vi "Skipback_171213.vi"(6 "Y out 3":i32[](array[numeric]), 9 "X in":i32[](array[numeric]), 10 "Skip Back Button":bool, 11 "Boolean in":refnum<vi>) -> (2 "Y out":i32[](array[numeric]), 3 "Y out 2":i32[](array[numeric]))   [LabVIEW 2016]
uses:
  Globaltracker.vi
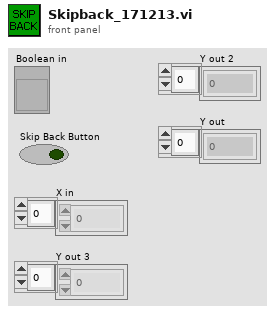
[diagram p1: front panel]
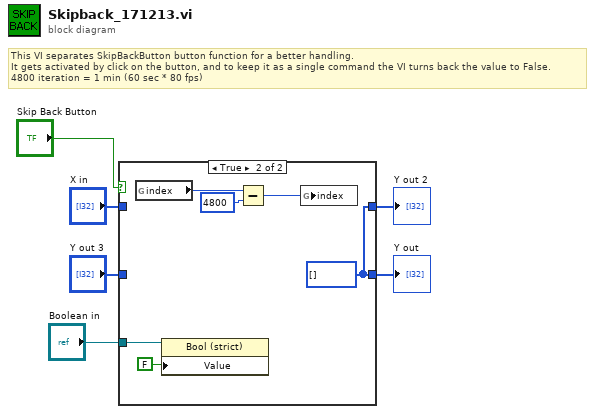
[diagram p0: block diagram]
diagram:
  # "This VI separates SkipBackButton button function for a better handling.\nIt gets activated by click on the button, and to keep it as a single command the VI turns back the value to False. \n4800 iteration = 1 min (60 sec * 80 fps)"
  n1 = case shown="True" "Skip Back Button" {
    tunnel: [w8 w12] -> w4
    tunnel: [w7 w12] -> w5
    tunnel: "X in" -> [w8 _]
    tunnel: "Y out 3" -> [w7 _]
    tunnel: "Boolean in" -> [_ w9]
    frame False {
    }
    frame True {
      w12 = i32[] [] ("Y out")
      n2 = global read "Globaltracker.vi" "index"() -> (w11:i16)
      n3 = property class="Bool (strict)"(reference=w9, "Value"=FALSE ("Skip Forward Button")) -> ()  [unwired: 1 in, 2 out]
      n4 = Subtract(x=w11, y=4800) -> (x-y=w10:i32)
      n5 = global write "Globaltracker.vi" "index"(w10) -> ()
    }
  }
  "Y out" <- w5
  "Y out 2" <- w4
